vi "Actor Core.vi"(8 "error in":errorcluster, 11 "User Interface":refnum<class "Client UI.lvclass">) -> (0 "error out":errorcluster, 3 "Actor out":refnum<class "Actor.lvclass">)   [LabVIEW 2026, in "Client UI.lvlib" / "Client UI.lvclass"]
doc: "This is Actor Core.vi, the main message handling loop for Actors. An actor usually just sits in this loop and processes messages as they arrive. Any error returned by the message Do.vi call will stop the loop, with error code 43 as the cannonical signal to stop with no error sent to caller. Descendants may override that in Handle Error.vi."
uses:
  Client UI.lvclass
  Client UI.lvclass/Client UI.ctl
  C:/Users/E2013170/Documents/GitHub/Measurement-Utility-Reference/components/MAL-Framework/user.lib/Common Components/Msmt UI/Measurement UI.lvclass
  C:/Users/E2013170/Documents/GitHub/Measurement-Utility-Reference/components/MAL-Framework/user.lib/Common Components/User Interface/UI.lvclass
  C:/Program Files/National Instruments/LabVIEW 2026/vi.lib/ActorFramework/Actor/Actor.lvclass
  C:/Users/E2013170/Documents/GitHub/Measurement-Utility-Reference/components/HAL-MAL-Application/Source/Framework/Client/UI/Client UI.lvclass
  MAL-Framework/user.lib/Common Components/User Interface/UI.lvclass
  <vilib>/ActorFramework/Actor/Actor.lvclass
  <vilib>/ActorFramework/Stop Msg/Stop Msg.lvclass
  MAL-Framework/user.lib/Common Components/Msmt UI/Messages/Tell Controller to Launch Settings Dialog Msg/Tell Controller to Launch Settings Dialog Msg.lvclass
  MAL-Framework/user.lib/Common Components/Msmt UI/Measurement UI.lvclass
panel:
  out "String":string
  in  "Settings Button":bool
  in  "Stop Button":bool
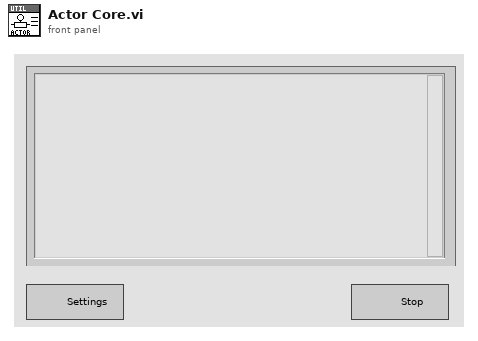
[diagram p1: front panel]
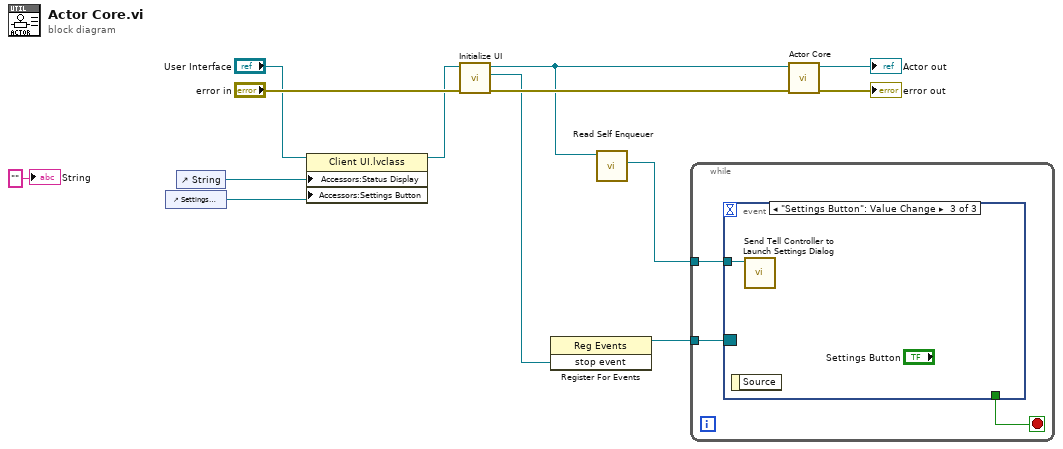
[diagram p0: block diagram]
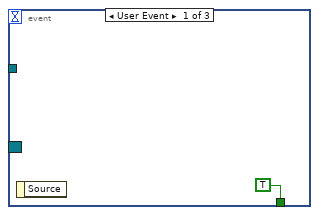
[diagram p2: hidden frame]
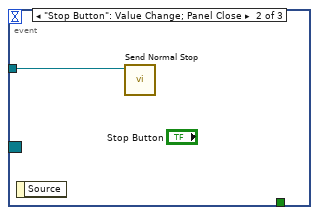
[diagram p3: hidden frame]
diagram:
  n1 = control-ref of="Settings Button"() -> (w2:refnum<vi>)
  n2 = control-ref of="String"() -> (w3:refnum<vi>)
  n3 = property class="Client UI.lvclass"(reference="User Interface", "Accessors:Status Display"=w3, "Accessors:Settings Button"=w2) -> (reference out=w4:refnum<class "Client UI.lvclass">)  [unwired: 1 in, 1 out]
  n4 = call "Initialize UI.vi"("error in (no error)"="error in", "UI in"=w4) -> ("error out"=w11:errorcluster, "stop event"=w10:refnum<user-event>, "UI out"=w1:refnum<class "Client UI.lvclass">)  [unwired: 7 in]
  n5 = register-events(w10) -> (reference out=w8:refnum<event-registration>)  [unwired: 2 in, 1 out]
  n6 = call <vilib>:"Read Self Enqueuer.vi"("Actor"=w1) -> ("Self Enqueuer"=w9:refnum<class "Message Enqueuer.lvclass">)  [unwired: 10 in]
  n7 = while {
    tunnel: w9 -> [w16]
    tunnel: w8 -> [w14]
    stop <- w15 stop-if-true
    n8 = event shown="[2] \"Settings Button\": Value Change" {
      selector: w14 -> [_ _ _]
      dyn-events: _ -> [_ _ _]
      timeout: _ -> [_ _ _]
      tunnel: w16 -> [_ w18 w19]
      tunnel: [TRUE _ _] -> w15
      event User Event {
        n9 = event-data() -> ()  [unwired: 1 in, 1 out]
      }
      event "Stop Button": Value Change; Panel Close {
        n10 = event-data() -> ()  [unwired: 1 in, 1 out]
        n11 = call <vilib>:"Send Normal Stop.vi"("Message Enqueuer"=w18) -> ()  [unwired: 10 in, 1 out]
      }
      event "Settings Button": Value Change {
        n12 = event-data() -> ()  [unwired: 1 in, 1 out]
        n13 = call "Send Tell Controller to Launch Settings Dialog.vi"("Message Enqueuer"=w19) -> ()  [unwired: 9 in, 2 out]
      }
    }
  }
  n14 = call-parent "Actor Core.vi"("error in (no error)"=w11, "Operator UI.lvclass"=w1) -> ("error out"=→"error out":errorcluster, "Actor Framework.lvlib:Actor"=→"Actor out":refnum<class "Actor.lvclass">)  [unwired: 8 in]
  "String" <- "" ("String")
